vi "TEST - Sort Array.vi"(8 "error in (no error)":errorcluster) -> (0 "error out":errorcluster, 2 "Pass?":bool=TRUE)   [LabVIEW 2020]
doc: "This VI template can be used for the functional testing of VIs; this implementation includes handling for the testing of polymorphic VIs, and the polymorphic elements should be removed if not needed.\n\nCoded by Douglas A. Femec, January 24, 2006.\n\nCopyright (c) 2005-2006 MKS Instruments, Inc.\nAll rights reserved."
uses:
  TEST - Sort Array - Inputs.ctl
  Polymorphizer+ Data Type.ctl
  TEST - Sort Array - Outputs.ctl
  source/library/Sort Array/Sort 2D Array (EXT).vi
  source/library/Sort Array/Sort 1D Array (EXT).vi
  source/library/Sort Array/Sort 2D Array (DBL).vi
  source/library/Sort Array/Sort 1D Array (DBL).vi
  source/library/Sort Array/Sort 2D Array (SGL).vi
  source/library/Sort Array/Sort 1D Array (SGL).vi
  source/library/Sort Array/Sort 2D Array (I32).vi
  source/library/Sort Array/Sort 1D Array (I32).vi
  source/library/Sort Array/Sort 2D Array (I16).vi
  source/library/Sort Array/Sort 1D Array (I16).vi
  source/library/Sort Array/Sort 2D Array (I8).vi
  source/library/Sort Array/Sort 1D Array (I8).vi
  source/library/Sort Array/Sort 2D Array (I64).vi
  source/library/Sort Array/Sort 1D Array (I64).vi
  source/library/Sort Array/Sort 2D Array (U64).vi
  source/library/Sort Array/Sort 1D Array (U64).vi
  source/library/Sort Array/Sort 2D Array (U32).vi
  source/library/Sort Array/Sort 1D Array (U32).vi
  source/library/Sort Array/Sort 2D Array (U16).vi
  source/library/Sort Array/Sort 1D Array (U16).vi
  source/library/Sort Array/Sort 2D Array (U8).vi
  source/library/Sort Array/Sort 1D Array (U8).vi
  source/library/Sort Array/Sort 2D Array (CXT).vi
  source/library/Sort Array/Sort 1D Array (CXT).vi
  source/library/Sort Array/Sort 2D Array (CDB).vi
  source/library/Sort Array/Sort 1D Array (CDB).vi
  source/library/Sort Array/Sort 2D Array (CSG).vi
  source/library/Sort Array/Sort 1D Array (CSG).vi
  source/library/Sort Array/Sort 2D Array (String).vi
  source/library/Sort Array/Sort 1D Array (String).vi
  source/library/Sort Array/Sort 2D Array (Path).vi
  source/library/Sort Array/Sort 1D Array (Path).vi
  source/library/openg_array.lvlib
panel:
  out "Generated Outputs":T1[][](array[typedef]) {"1D Array" format="%.2f"; "2D Array" format="%.2f"}
  in  "Expected Outputs":T1[](array[typedef])=[{"Description"="Expect empty arrays", "1D Array"=[], "2D Array"=[], "1D Sorted Pointers"=[], "2D Sorted Pointers"=[], "Index Out of Range?"=FALSE, "Sort By in"=enum."row"}, {"Description"="Expect empty arrays", "1D Array"=[], "2D Array"=[], "1D Sorted Pointers"=[], "2D Sorted Pointers"=[], "Index Out of Range?"=FALSE, "Sort By in"=enum."row"}, {"Description"="Expect empty arrays", "1D Array"=[], "2D Array"=[], "1D Sorted Pointers"=[], "2D Sorted Pointers"=[], "Index Out of Range?"=FALSE, "Sort By in"=enum."row"}, {"Description"="Expect empty arrays", "1D Array"=[], "2D Array"=[], "1D Sorted Pointers"=[], "2D Sorted Pointers"=[], "Index Out of Range?"=FALSE, "Sort By in"=enum."column"}, {"Description"="Expect empty arrays", "1D Array"=[], "2D Array"=[], "1D Sorted Pointers"=[], "2D Sorted Pointers"=[], "Index Out of Range?"=FALSE, "Sort By in"=enum."column"}, {"Description"="Expect empty arrays", "1D Array"=[], "2D Array"=[], "1D Sorted Pointers"=[], "2D Sorted Pointers"=[], "Index Out of Range?"=FALSE, "Sort By in"=enum."column"}, {"Description"="Expect empty arrays", "1D Array"=[], "2D Array"=[], "1D Sorted Pointers"=[], "2D Sorted Pointers"=[], "Index Out of Range?"=FALSE, "Sort By in"=enum."row"}, {"Description"="Expect empty arrays", "1D Array"=[], "2D Array"=[], "1D Sorted Pointers"=[], "2D Sorted Pointers"=[], "Index Out of Range?"=FALSE, "Sort By in"=enum."row"}, {"Description"="Expect empty arrays", "1D Array"=[], "2D Array"=[], "1D Sorted Pointers"=[], "2D Sorted Pointers"=[], "Index Out of Range?"=FALSE, "Sort By in"=enum."row"}, {"Description"="Expect empty arrays", "1D Array"=[], "2D Array"=[], "1D Sorted Pointers"=[], "2D Sorted Pointers"=[], "Index Out of Range?"=FALSE, "Sort By in"=enum."column"}, {"Description"="Expect empty arrays", "1D Array"=[], "2D Array"=[], "1D Sorted Pointers"=[], "2D Sorted Pointers"=[], "Index Out of Range?"=FALSE, "Sort By in"=enum."column"}, {"Description"="Expect empty arrays", "1D Array"=[], "2D Array"=[], "1D Sorted Pointers"=[], "2D Sorted Pointers"=[], "Index Out of Range?"=FALSE, "Sort By in"=enum."column"}, {"Description"="Expect sorted in ascending order, 2D by row 0", "1D Array"=[0.0, 1.0, 2.0, 3.0, 4.0], "2D Array"=[[0.0, 5.0], [1.0, 6.0], [2.0, 7.0], [3.0, 8.0], [4.0, 9.0]], "1D Sorted Pointers"=[0, 1, 2, 3, 4], "2D Sorted Pointers"=[0, 1], "Index Out of Range?"=FALSE, "Sort By in"=enum."row"}, {"Description"="Expect sorted in ascending order, 2D by row 1", "1D Array"=[0.0, 1.0, 2.0, 3.0, 4.0], "2D Array"=[[0.0, 5.0], [1.0, 6.0], [2.0, 7.0], [3.0, 8.0], [4.0, 9.0]], "1D Sorted Pointers"=[0, 1, 2, 3, 4], "2D Sorted Pointers"=[0, 1], "Index Out of Range?"=FALSE, "Sort By in"=enum."row"}, {"Description"="Expect sorted in ascending order, 2D no row 5, so expect index out of range", "1D Array"=[0.0, 1.0, 2.0, 3.0, 4.0], "2D Array"=[], "1D Sorted Pointers"=[0, 1, 2, 3, 4], "2D Sorted Pointers"=[], "Index Out of Range?"=TRUE, "Sort By in"=enum."row"}, {"Description"="Expect sorted in ascending order, 2D by column 0", "1D Array"=[0.0, 1.0, 2.0, 3.0, 4.0], "2D Array"=[[0.0, 5.0], [1.0, 6.0], [2.0, 7.0], [3.0, 8.0], [4.0, 9.0]], "1D Sorted Pointers"=[0, 1, 2, 3, 4], "2D Sorted Pointers"=[0, 1, 2, 3, 4], "Index Out of Range?"=FALSE, "Sort By in"=enum."column"}, {"Description"="Expect sorted in ascending order, 2D by column 1", "1D Array"=[0.0, 1.0, 2.0, 3.0, 4.0], "2D Array"=[[0.0, 5.0], [1.0, 6.0], [2.0, 7.0], [3.0, 8.0], [4.0, 9.0]], "1D Sorted Pointers"=[0, 1, 2, 3, 4], "2D Sorted Pointers"=[0, 1, 2, 3, 4], "Index Out of Range?"=FALSE, "Sort By in"=enum."column"}, {"Description"="Expect sorted in ascending order, 2D no column 5, so expect index out of range", "1D Array"=[0.0, 1.0, 2.0, 3.0, 4.0], "2D Array"=[], "1D Sorted Pointers"=[0, 1, 2, 3, 4], "2D Sorted Pointers"=[], "Index Out of Range?"=TRUE, "Sort By in"=enum."column"}, {"Description"="Expect sorted in descending order, 2D by row 0", "1D Array"=[4.0, 3.0, 2.0, 1.0, 0.0], "2D Array"=[[5.0, 0.0], [6.0, 1.0], [7.0, 2.0], [8.0, 3.0], [9.0, 4.0]], "1D Sorted Pointers"=[4, 3, 2, 1, 0], "2D Sorted Pointers"=[1, 0], "Index Out of Range?"=FALSE, "Sort By in"=enum."row"}, {"Description"="Expect sorted in descending order, 2D by row 1", "1D Array"=[4.0, 3.0, 2.0, 1.0, 0.0], "2D Array"=[[5.0, 0.0], [6.0, 1.0], [7.0, 2.0], [8.0, 3.0], [9.0, 4.0]], "1D Sorted Pointers"=[4, 3, 2, 1, 0], "2D Sorted Pointers"=[1, 0], "Index Out of Range?"=FALSE, "Sort By in"=enum."row"}, {"Description"="Expect sorted in descending order, 2D no row 5, so expect index out of range", "1D Array"=[4.0, 3.0, 2.0, 1.0, 0.0], "2D Array"=[], "1D Sorted Pointers"=[4, 3, 2, 1, 0], "2D Sorted Pointers"=[], "Index Out of Range?"=TRUE, "Sort By in"=enum."row"}, {"Description"="Expect sorted in descending order, 2D by column 0", "1D Array"=[4.0, 3.0, 2.0, 1.0, 0.0], "2D Array"=[[4.0, 9.0], [3.0, 8.0], [2.0, 7.0], [1.0, 6.0], [0.0, 5.0]], "1D Sorted Pointers"=[4, 3, 2, 1, 0], "2D Sorted Pointers"=[4, 3, 2, 1, 0], "Index Out of Range?"=FALSE, "Sort By in"=enum."column"}, {"Description"="Expect sorted in descending order, 2D by column 1", "1D Array"=[4.0, 3.0, 2.0, 1.0, 0.0], "2D Array"=[[4.0, 9.0], [3.0, 8.0], [2.0, 7.0], [1.0, 6.0], [0.0, 5.0]], "1D Sorted Pointers"=[4, 3, 2, 1, 0], "2D Sorted Pointers"=[4, 3, 2, 1, 0], "Index Out of Range?"=FALSE, "Sort By in"=enum."column"}, {"Description"="Expect sorted in descending order, 2D no column 5, so expect index out of range", "1D Array"=[4.0, 3.0, 2.0, 1.0, 0.0], "2D Array"=[], "1D Sorted Pointers"=[4, 3, 2, 1, 0], "2D Sorted Pointers"=[], "Index Out of Range?"=TRUE, "Sort By in"=enum."column"}, {"Description"="Expect sorted in ascending order, 2D by row 0", "1D Array"=[0.0, 1.0, 2.0, 3.0, 4.0], "2D Array"=[[4.0, 9.0], [3.0, 8.0], [2.0, 7.0], [1.0, 6.0], [0.0, 5.0]], "1D Sorted Pointers"=[4, 3, 2, 1, 0], "2D Sorted Pointers"=[1, 0], "Index Out of Range?"=FALSE, "Sort By in"=enum."row"}, {"Description"="Expect sorted in ascending order, 2D by row 1", "1D Array"=[0.0, 1.0, 2.0, 3.0, 4.0], "2D Array"=[[4.0, 9.0], [3.0, 8.0], [2.0, 7.0], [1.0, 6.0], [0.0, 5.0]], "1D Sorted Pointers"=[4, 3, 2, 1, 0], "2D Sorted Pointers"=[1, 0], "Index Out of Range?"=FALSE, "Sort By in"=enum."row"}, {"Description"="Expect sorted in ascending order, 2D no row 5, so expect index out of range", "1D Array"=[0.0, 1.0, 2.0, 3.0, 4.0], "2D Array"=[], "1D Sorted Pointers"=[4, 3, 2, 1, 0], "2D Sorted Pointers"=[], "Index Out of Range?"=TRUE, "Sort By in"=enum."row"}, {"Description"="Expect sorted in descending order, 2D by column 0", "1D Array"=[0.0, 1.0, 2.0, 3.0, 4.0], "2D Array"=[[5.0, 0.0], [6.0, 1.0], [7.0, 2.0], [8.0, 3.0], [9.0, 4.0]], "1D Sorted Pointers"=[4, 3, 2, 1, 0], "2D Sorted Pointers"=[4, 3, 2, 1, 0], "Index Out of Range?"=FALSE, "Sort By in"=enum."column"}, {"Description"="Expect sorted in descending order, 2D by column 1", "1D Array"=[0.0, 1.0, 2.0, 3.0, 4.0], "2D Array"=[[5.0, 0.0], [6.0, 1.0], [7.0, 2.0], [8.0, 3.0], [9.0, 4.0]], "1D Sorted Pointers"=[4, 3, 2, 1, 0], "2D Sorted Pointers"=[4, 3, 2, 1, 0], "Index Out of Range?"=FALSE, "Sort By in"=enum."column"}, {"Description"="Expect sorted in descending order, 2D no column 5, so expect index out of range", "1D Array"=[0.0, 1.0, 2.0, 3.0, 4.0], "2D Array"=[], "1D Sorted Pointers"=[4, 3, 2, 1, 0], "2D Sorted Pointers"=[], "Index Out of Range?"=TRUE, "Sort By in"=enum."column"}, {"Description"="Expect sorted in descending order, 2D by row 0", "1D Array"=[4.0, 3.0, 2.0, 1.0, 0.0], "2D Array"=[[9.0, 4.0], [8.0, 3.0], [7.0, 2.0], [6.0, 1.0], [5.0, 0.0]], "1D Sorted Pointers"=[0, 1, 2, 3, 4], "2D Sorted Pointers"=[0, 1], "Index Out of Range?"=FALSE, "Sort By in"=enum."row"}, {"Description"="Expect sorted in descending order, 2D by row 1", "1D Array"=[4.0, 3.0, 2.0, 1.0, 0.0], "2D Array"=[[9.0, 4.0], [8.0, 3.0], [7.0, 2.0], [6.0, 1.0], [5.0, 0.0]], "1D Sorted Pointers"=[0, 1, 2, 3, 4], "2D Sorted Pointers"=[0, 1], "Index Out of Range?"=FALSE, "Sort By in"=enum."row"}, {"Description"="Expect sorted in descending order, 2D no row 5, so expect index out of range", "1D Array"=[4.0, 3.0, 2.0, 1.0, 0.0], "2D Array"=[], "1D Sorted Pointers"=[0, 1, 2, 3, 4], "2D Sorted Pointers"=[], "Index Out of Range?"=TRUE, "Sort By in"=enum."row"}, {"Description"="Expect sorted in descending order, 2D by column 0", "1D Array"=[4.0, 3.0, 2.0, 1.0, 0.0], "2D Array"=[[9.0, 4.0], [8.0, 3.0], [7.0, 2.0], [6.0, 1.0], [5.0, 0.0]], "1D Sorted Pointers"=[0, 1, 2, 3, 4], "2D Sorted Pointers"=[0, 1, 2, 3, 4], "Index Out of Range?"=FALSE, "Sort By in"=enum."column"}, {"Description"="Expect sorted in descending order, 2D by column 1", "1D Array"=[4.0, 3.0, 2.0, 1.0, 0.0], "2D Array"=[[9.0, 4.0], [8.0, 3.0], [7.0, 2.0], [6.0, 1.0], [5.0, 0.0]], "1D Sorted Pointers"=[0, 1, 2, 3, 4], "2D Sorted Pointers"=[0, 1, 2, 3, 4], "Index Out of Range?"=FALSE, "Sort By in"=enum."column"}, {"Description"="Expect sorted in descending order, 2D no column 5, so expect index out of range", "1D Array"=[4.0, 3.0, 2.0, 1.0, 0.0], "2D Array"=[], "1D Sorted Pointers"=[0, 1, 2, 3, 4], "2D Sorted Pointers"=[], "Index Out of Range?"=TRUE, "Sort By in"=enum."column"}, {"Description"="Expect sorted in ascending order, 2D by row 0", "1D Array"=[0.0, 1.0, 2.0, 3.0, 4.0], "2D Array"=[[3.0, 6.0], [2.0, 9.0], [0.0, 5.0], [4.0, 7.0], [1.0, 8.0]], "1D Sorted Pointers"=[2, 4, 1, 0, 3], "2D Sorted Pointers"=[0, 1], "Index Out of Range?"=FALSE, "Sort By in"=enum."row"}, {"Description"="Expect sorted in ascending order, 2D by row 1", "1D Array"=[0.0, 1.0, 2.0, 3.0, 4.0], "2D Array"=[[3.0, 6.0], [2.0, 9.0], [0.0, 5.0], [4.0, 7.0], [1.0, 8.0]], "1D Sorted Pointers"=[2, 4, 1, 0, 3], "2D Sorted Pointers"=[0, 1], "Index Out of Range?"=FALSE, "Sort By in"=enum."row"}, {"Description"="Expect sorted in ascending order, 2D no row 5, so expect index out of range", "1D Array"=[0.0, 1.0, 2.0, 3.0, 4.0], "2D Array"=[], "1D Sorted Pointers"=[2, 4, 1, 0, 3], "2D Sorted Pointers"=[], "Index Out of Range?"=TRUE, "Sort By in"=enum."row"}, {"Description"="Expect sorted in ascending order, 2D by column 0", "1D Array"=[0.0, 1.0, 2.0, 3.0, 4.0], "2D Array"=[[0.0, 5.0], [1.0, 8.0], [2.0, 9.0], [3.0, 6.0], [4.0, 7.0]], "1D Sorted Pointers"=[2, 4, 1, 0, 3], "2D Sorted Pointers"=[2, 4, 1, 0, 3], "Index Out of Range?"=FALSE, "Sort By in"=enum."column"}, {"Description"="Expect sorted in ascending order, 2D by column 1", "1D Array"=[0.0, 1.0, 2.0, 3.0, 4.0], "2D Array"=[[0.0, 5.0], [3.0, 6.0], [4.0, 7.0], [1.0, 8.0], [2.0, 9.0]], "1D Sorted Pointers"=[2, 4, 1, 0, 3], "2D Sorted Pointers"=[2, 0, 3, 4, 1], "Index Out of Range?"=FALSE, "Sort By in"=enum."column"}, {"Description"="Expect sorted in ascending order, 2D no column 5, so expect index out of range", "1D Array"=[0.0, 1.0, 2.0, 3.0, 4.0], "2D Array"=[], "1D Sorted Pointers"=[2, 4, 1, 0, 3], "2D Sorted Pointers"=[], "Index Out of Range?"=TRUE, "Sort By in"=enum."column"}, {"Description"="Expect sorted in descending order, 2D by row 0", "1D Array"=[4.0, 3.0, 2.0, 1.0, 0.0], "2D Array"=[[6.0, 3.0], [9.0, 2.0], [5.0, 0.0], [7.0, 4.0], [8.0, 1.0]], "1D Sorted Pointers"=[3, 0, 1, 4, 2], "2D Sorted Pointers"=[1, 0], "Index Out of Range?"=FALSE, "Sort By in"=enum."row"}, {"Description"="Expect sorted in descending order, 2D by row 1", "1D Array"=[4.0, 3.0, 2.0, 1.0, 0.0], "2D Array"=[[6.0, 3.0], [9.0, 2.0], [5.0, 0.0], [7.0, 4.0], [8.0, 1.0]], "1D Sorted Pointers"=[3, 0, 1, 4, 2], "2D Sorted Pointers"=[1, 0], "Index Out of Range?"=FALSE, "Sort By in"=enum."row"}, {"Description"="Expect sorted in descending order, 2D no row 5, so expect index out of range", "1D Array"=[4.0, 3.0, 2.0, 1.0, 0.0], "2D Array"=[], "1D Sorted Pointers"=[3, 0, 1, 4, 2], "2D Sorted Pointers"=[], "Index Out of Range?"=TRUE, "Sort By in"=enum."row"}, {"Description"="Expect sorted in descending order, 2D by column 0", "1D Array"=[4.0, 3.0, 2.0, 1.0, 0.0], "2D Array"=[[4.0, 7.0], [3.0, 6.0], [2.0, 9.0], [1.0, 8.0], [0.0, 5.0]], "1D Sorted Pointers"=[3, 0, 1, 4, 2], "2D Sorted Pointers"=[3, 0, 1, 4, 2], "Index Out of Range?"=FALSE, "Sort By in"=enum."column"}, {"Description"="Expect sorted in descending order, 2D by column 1", "1D Array"=[4.0, 3.0, 2.0, 1.0, 0.0], "2D Array"=[[2.0, 9.0], [1.0, 8.0], [4.0, 7.0], [3.0, 6.0], [0.0, 5.0]], "1D Sorted Pointers"=[3, 0, 1, 4, 2], "2D Sorted Pointers"=[1, 4, 3, 0, 2], "Index Out of Range?"=FALSE, "Sort By in"=enum."column"}, {"Description"="Expect sorted in ascending order, 2D no column 5, so expect index out of range", "1D Array"=[4.0, 3.0, 2.0, 1.0, 0.0], "2D Array"=[], "1D Sorted Pointers"=[3, 0, 1, 4, 2], "2D Sorted Pointers"=[], "Index Out of Range?"=TRUE, "Sort By in"=enum."column"}] {"1D Array" format="%.2f"; "2D Array" format="%.2f"}
  in  "Inputs":T2[](array[typedef])=[{"Description"="Empty arrays, ascending, 2D by row 0", "Data Types to Test"=[enum."EXT", enum."DBL", enum."SGL", enum."I32", enum."I16", enum."I8", enum."U32", enum."U16", enum."U8", enum."CXT", enum."CDB", enum."CSG", enum."String", enum."Path", enum."I64", enum."U64"], "1D Array"=[], "2D Array"=[], "Order"=enum."ascending", "Sort By in"=enum."row", "Column/Row to Sort By"=0}, {"Description"="Empty arrays, ascending, 2D by row 1", "Data Types to Test"=[enum."EXT", enum."DBL", enum."SGL", enum."I32", enum."I16", enum."I8", enum."U32", enum."U16", enum."U8", enum."CXT", enum."CDB", enum."CSG", enum."String", enum."Path", enum."I64", enum."U64"], "1D Array"=[], "2D Array"=[], "Order"=enum."ascending", "Sort By in"=enum."row", "Column/Row to Sort By"=1}, {"Description"="Empty arrays, ascending, 2D by row 5", "Data Types to Test"=[enum."EXT", enum."DBL", enum."SGL", enum."I32", enum."I16", enum."I8", enum."U32", enum."U16", enum."U8", enum."CXT", enum."CDB", enum."CSG", enum."String", enum."Path", enum."I64", enum."U64"], "1D Array"=[], "2D Array"=[], "Order"=enum."ascending", "Sort By in"=enum."row", "Column/Row to Sort By"=5}, {"Description"="Empty arrays, ascending, 2D by column 0", "Data Types to Test"=[enum."EXT", enum."DBL", enum."SGL", enum."I32", enum."I16", enum."I8", enum."U32", enum."U16", enum."U8", enum."CXT", enum."CDB", enum."CSG", enum."String", enum."Path", enum."I64", enum."U64"], "1D Array"=[], "2D Array"=[], "Order"=enum."ascending", "Sort By in"=enum."column", "Column/Row to Sort By"=0}, {"Description"="Empty arrays, ascending, 2D by column 1", "Data Types to Test"=[enum."EXT", enum."DBL", enum."SGL", enum."I32", enum."I16", enum."I8", enum."U32", enum."U16", enum."U8", enum."CXT", enum."CDB", enum."CSG", enum."String", enum."Path", enum."I64", enum."U64"], "1D Array"=[], "2D Array"=[], "Order"=enum."ascending", "Sort By in"=enum."column", "Column/Row to Sort By"=1}, {"Description"="Empty arrays, ascending, 2D by column 5", "Data Types to Test"=[enum."EXT", enum."DBL", enum."SGL", enum."I32", enum."I16", enum."I8", enum."U32", enum."U16", enum."U8", enum."CXT", enum."CDB", enum."CSG", enum."String", enum."Path", enum."I64", enum."U64"], "1D Array"=[], "2D Array"=[], "Order"=enum."ascending", "Sort By in"=enum."column", "Column/Row to Sort By"=5}, {"Description"="Empty arrays, descending, 2D by row 0", "Data Types to Test"=[enum."EXT", enum."DBL", enum."SGL", enum."I32", enum."I16", enum."I8", enum."U32", enum."U16", enum."U8", enum."CXT", enum."CDB", enum."CSG", enum."String", enum."Path", enum."I64", enum."U64"], "1D Array"=[], "2D Array"=[], "Order"=enum."descending", "Sort By in"=enum."row", "Column/Row to Sort By"=0}, {"Description"="Empty arrays, descending, 2D by row 1", "Data Types to Test"=[enum."EXT", enum."DBL", enum."SGL", enum."I32", enum."I16", enum."I8", enum."U32", enum."U16", enum."U8", enum."CXT", enum."CDB", enum."CSG", enum."String", enum."Path", enum."I64", enum."U64"], "1D Array"=[], "2D Array"=[], "Order"=enum."descending", "Sort By in"=enum."row", "Column/Row to Sort By"=1}, {"Description"="Empty arrays, descending, 2D by row 5", "Data Types to Test"=[enum."EXT", enum."DBL", enum."SGL", enum."I32", enum."I16", enum."I8", enum."U32", enum."U16", enum."U8", enum."CXT", enum."CDB", enum."CSG", enum."String", enum."Path", enum."I64", enum."U64"], "1D Array"=[], "2D Array"=[], "Order"=enum."descending", "Sort By in"=enum."row", "Column/Row to Sort By"=5}, {"Description"="Empty arrays, descending, 2D by column 0", "Data Types to Test"=[enum."EXT", enum."DBL", enum."SGL", enum."I32", enum."I16", enum."I8", enum."U32", enum."U16", enum."U8", enum."CXT", enum."CDB", enum."CSG", enum."String", enum."Path", enum."I64", enum."U64"], "1D Array"=[], "2D Array"=[], "Order"=enum."descending", "Sort By in"=enum."column", "Column/Row to Sort By"=0}, {"Description"="Empty arrays, descending, 2D by column 1", "Data Types to Test"=[enum."EXT", enum."DBL", enum."SGL", enum."I32", enum."I16", enum."I8", enum."U32", enum."U16", enum."U8", enum."CXT", enum."CDB", enum."CSG", enum."String", enum."Path", enum."I64", enum."U64"], "1D Array"=[], "2D Array"=[], "Order"=enum."descending", "Sort By in"=enum."column", "Column/Row to Sort By"=1}, {"Description"="Empty arrays, descending, 2D by column 5", "Data Types to Test"=[enum."EXT", enum."DBL", enum."SGL", enum."I32", enum."I16", enum."I8", enum."U32", enum."U16", enum."U8", enum."CXT", enum."CDB", enum."CSG", enum."String", enum."Path", enum."I64", enum."U64"], "1D Array"=[], "2D Array"=[], "Order"=enum."descending", "Sort By in"=enum."column", "Column/Row to Sort By"=5}, {"Description"="Already sorted in ascending order, ascending, 2D by row 0", "Data Types to Test"=[enum."EXT", enum."DBL", enum."SGL", enum."I32", enum."I16", enum."I8", enum."U32", enum."U16", enum."U8", enum."CXT", enum."CDB", enum."CSG", enum."String", enum."Path", enum."I64", enum."U64"], "1D Array"=[0.0, 1.0, 2.0, 3.0, 4.0], "2D Array"=[[0.0, 5.0], [1.0, 6.0], [2.0, 7.0], [3.0, 8.0], [4.0, 9.0]], "Order"=enum."ascending", "Sort By in"=enum."row", "Column/Row to Sort By"=0}, {"Description"="Already sorted in ascending order, ascending, 2D by row 1", "Data Types to Test"=[enum."EXT", enum."DBL", enum."SGL", enum."I32", enum."I16", enum."I8", enum."U32", enum."U16", enum."U8", enum."CXT", enum."CDB", enum."CSG", enum."String", enum."Path", enum."I64", enum."U64"], "1D Array"=[0.0, 1.0, 2.0, 3.0, 4.0], "2D Array"=[[0.0, 5.0], [1.0, 6.0], [2.0, 7.0], [3.0, 8.0], [4.0, 9.0]], "Order"=enum."ascending", "Sort By in"=enum."row", "Column/Row to Sort By"=1}, {"Description"="Already sorted in ascending order, ascending, 2D by row 5", "Data Types to Test"=[enum."EXT", enum."DBL", enum."SGL", enum."I32", enum."I16", enum."I8", enum."U32", enum."U16", enum."U8", enum."CXT", enum."CDB", enum."CSG", enum."String", enum."Path", enum."I64", enum."U64"], "1D Array"=[0.0, 1.0, 2.0, 3.0, 4.0], "2D Array"=[[0.0, 5.0], [1.0, 6.0], [2.0, 7.0], [3.0, 8.0], [4.0, 9.0]], "Order"=enum."ascending", "Sort By in"=enum."row", "Column/Row to Sort By"=5}, {"Description"="Already sorted in ascending order, ascending, 2D by column 0", "Data Types to Test"=[enum."EXT", enum."DBL", enum."SGL", enum."I32", enum."I16", enum."I8", enum."U32", enum."U16", enum."U8", enum."CXT", enum."CDB", enum."CSG", enum."String", enum."Path", enum."I64", enum."U64"], "1D Array"=[0.0, 1.0, 2.0, 3.0, 4.0], "2D Array"=[[0.0, 5.0], [1.0, 6.0], [2.0, 7.0], [3.0, 8.0], [4.0, 9.0]], "Order"=enum."ascending", "Sort By in"=enum."column", "Column/Row to Sort By"=0}, {"Description"="Already sorted in ascending order, ascending, 2D by column 1", "Data Types to Test"=[enum."EXT", enum."DBL", enum."SGL", enum."I32", enum."I16", enum."I8", enum."U32", enum."U16", enum."U8", enum."CXT", enum."CDB", enum."CSG", enum."String", enum."Path", enum."I64", enum."U64"], "1D Array"=[0.0, 1.0, 2.0, 3.0, 4.0], "2D Array"=[[0.0, 5.0], [1.0, 6.0], [2.0, 7.0], [3.0, 8.0], [4.0, 9.0]], "Order"=enum."ascending", "Sort By in"=enum."column", "Column/Row to Sort By"=1}, {"Description"="Already sorted in ascending order, ascending, 2D by column 5", "Data Types to Test"=[enum."EXT", enum."DBL", enum."SGL", enum."I32", enum."I16", enum."I8", enum."U32", enum."U16", enum."U8", enum."CXT", enum."CDB", enum."CSG", enum."String", enum."Path", enum."I64", enum."U64"], "1D Array"=[0.0, 1.0, 2.0, 3.0, 4.0], "2D Array"=[[0.0, 5.0], [1.0, 6.0], [2.0, 7.0], [3.0, 8.0], [4.0, 9.0]], "Order"=enum."ascending", "Sort By in"=enum."column", "Column/Row to Sort By"=5}, {"Description"="Already sorted in ascending order, descending, 2D by row 0", "Data Types to Test"=[enum."EXT", enum."DBL", enum."SGL", enum."I32", enum."I16", enum."I8", enum."U32", enum."U16", enum."U8", enum."CXT", enum."CDB", enum."CSG", enum."String", enum."Path", enum."I64", enum."U64"], "1D Array"=[0.0, 1.0, 2.0, 3.0, 4.0], "2D Array"=[[0.0, 5.0], [1.0, 6.0], [2.0, 7.0], [3.0, 8.0], [4.0, 9.0]], "Order"=enum."descending", "Sort By in"=enum."row", "Column/Row to Sort By"=0}, {"Description"="Already sorted in ascending order, descending, 2D by row 1", "Data Types to Test"=[enum."EXT", enum."DBL", enum."SGL", enum."I32", enum."I16", enum."I8", enum."U32", enum."U16", enum."U8", enum."CXT", enum."CDB", enum."CSG", enum."String", enum."Path", enum."I64", enum."U64"], "1D Array"=[0.0, 1.0, 2.0, 3.0, 4.0], "2D Array"=[[0.0, 5.0], [1.0, 6.0], [2.0, 7.0], [3.0, 8.0], [4.0, 9.0]], "Order"=enum."descending", "Sort By in"=enum."row", "Column/Row to Sort By"=1}, {"Description"="Already sorted in ascending order, descending, 2D by row 5", "Data Types to Test"=[enum."EXT", enum."DBL", enum."SGL", enum."I32", enum."I16", enum."I8", enum."U32", enum."U16", enum."U8", enum."CXT", enum."CDB", enum."CSG", enum."String", enum."Path", enum."I64", enum."U64"], "1D Array"=[0.0, 1.0, 2.0, 3.0, 4.0], "2D Array"=[[0.0, 5.0], [1.0, 6.0], [2.0, 7.0], [3.0, 8.0], [4.0, 9.0]], "Order"=enum."descending", "Sort By in"=enum."row", "Column/Row to Sort By"=5}, {"Description"="Already sorted in ascending order, descending, 2D by column 0", "Data Types to Test"=[enum."EXT", enum."DBL", enum."SGL", enum."I32", enum."I16", enum."I8", enum."U32", enum."U16", enum."U8", enum."CXT", enum."CDB", enum."CSG", enum."String", enum."Path", enum."I64", enum."U64"], "1D Array"=[0.0, 1.0, 2.0, 3.0, 4.0], "2D Array"=[[0.0, 5.0], [1.0, 6.0], [2.0, 7.0], [3.0, 8.0], [4.0, 9.0]], "Order"=enum."descending", "Sort By in"=enum."column", "Column/Row to Sort By"=0}, {"Description"="Already sorted in ascending order, descending, 2D by column 1", "Data Types to Test"=[enum."EXT", enum."DBL", enum."SGL", enum."I32", enum."I16", enum."I8", enum."U32", enum."U16", enum."U8", enum."CXT", enum."CDB", enum."CSG", enum."String", enum."Path", enum."I64", enum."U64"], "1D Array"=[0.0, 1.0, 2.0, 3.0, 4.0], "2D Array"=[[0.0, 5.0], [1.0, 6.0], [2.0, 7.0], [3.0, 8.0], [4.0, 9.0]], "Order"=enum."descending", "Sort By in"=enum."column", "Column/Row to Sort By"=1}, {"Description"="Already sorted in ascending order, descending, 2D by column 5", "Data Types to Test"=[enum."EXT", enum."DBL", enum."SGL", enum."I32", enum."I16", enum."I8", enum."U32", enum."U16", enum."U8", enum."CXT", enum."CDB", enum."CSG", enum."String", enum."Path", enum."I64", enum."U64"], "1D Array"=[0.0, 1.0, 2.0, 3.0, 4.0], "2D Array"=[[0.0, 5.0], [1.0, 6.0], [2.0, 7.0], [3.0, 8.0], [4.0, 9.0]], "Order"=enum."descending", "Sort By in"=enum."column", "Column/Row to Sort By"=5}, {"Description"="Already sorted in descending order, ascending, 2D by row 0", "Data Types to Test"=[enum."EXT", enum."DBL", enum."SGL", enum."I32", enum."I16", enum."I8", enum."U32", enum."U16", enum."U8", enum."CXT", enum."CDB", enum."CSG", enum."String", enum."Path", enum."I64", enum."U64"], "1D Array"=[4.0, 3.0, 2.0, 1.0, 0.0], "2D Array"=[[9.0, 4.0], [8.0, 3.0], [7.0, 2.0], [6.0, 1.0], [5.0, 0.0]], "Order"=enum."ascending", "Sort By in"=enum."row", "Column/Row to Sort By"=0}, {"Description"="Already sorted in descending order, ascending, 2D by row 1", "Data Types to Test"=[enum."EXT", enum."DBL", enum."SGL", enum."I32", enum."I16", enum."I8", enum."U32", enum."U16", enum."U8", enum."CXT", enum."CDB", enum."CSG", enum."String", enum."Path", enum."I64", enum."U64"], "1D Array"=[4.0, 3.0, 2.0, 1.0, 0.0], "2D Array"=[[9.0, 4.0], [8.0, 3.0], [7.0, 2.0], [6.0, 1.0], [5.0, 0.0]], "Order"=enum."ascending", "Sort By in"=enum."row", "Column/Row to Sort By"=1}, {"Description"="Already sorted in descending order, ascending, 2D by row 5", "Data Types to Test"=[enum."EXT", enum."DBL", enum."SGL", enum."I32", enum."I16", enum."I8", enum."U32", enum."U16", enum."U8", enum."CXT", enum."CDB", enum."CSG", enum."String", enum."Path", enum."I64", enum."U64"], "1D Array"=[4.0, 3.0, 2.0, 1.0, 0.0], "2D Array"=[[9.0, 4.0], [8.0, 3.0], [7.0, 2.0], [6.0, 2.0], [5.0, 1.0]], "Order"=enum."ascending", "Sort By in"=enum."row", "Column/Row to Sort By"=5}, {"Description"="Already sorted in descending order, ascending, 2D by column 0", "Data Types to Test"=[enum."EXT", enum."DBL", enum."SGL", enum."I32", enum."I16", enum."I8", enum."U32", enum."U16", enum."U8", enum."CXT", enum."CDB", enum."CSG", enum."String", enum."Path", enum."I64", enum."U64"], "1D Array"=[4.0, 3.0, 2.0, 1.0, 0.0], "2D Array"=[[9.0, 4.0], [8.0, 3.0], [7.0, 2.0], [6.0, 1.0], [5.0, 0.0]], "Order"=enum."ascending", "Sort By in"=enum."column", "Column/Row to Sort By"=0}, {"Description"="Already sorted in descending order, ascending, 2D by column 1", "Data Types to Test"=[enum."EXT", enum."DBL", enum."SGL", enum."I32", enum."I16", enum."I8", enum."U32", enum."U16", enum."U8", enum."CXT", enum."CDB", enum."CSG", enum."String", enum."Path", enum."I64", enum."U64"], "1D Array"=[4.0, 3.0, 2.0, 1.0, 0.0], "2D Array"=[[9.0, 4.0], [8.0, 3.0], [7.0, 2.0], [6.0, 1.0], [5.0, 0.0]], "Order"=enum."ascending", "Sort By in"=enum."column", "Column/Row to Sort By"=1}, {"Description"="Already sorted in descending order, ascending, 2D by column 5", "Data Types to Test"=[enum."EXT", enum."DBL", enum."SGL", enum."I32", enum."I16", enum."I8", enum."U32", enum."U16", enum."U8", enum."CXT", enum."CDB", enum."CSG", enum."String", enum."Path", enum."I64", enum."U64"], "1D Array"=[4.0, 3.0, 2.0, 1.0, 0.0], "2D Array"=[[9.0, 4.0], [8.0, 3.0], [7.0, 2.0], [6.0, 2.0], [5.0, 1.0]], "Order"=enum."ascending", "Sort By in"=enum."column", "Column/Row to Sort By"=5}, {"Description"="Already sorted in descending order, descending, 2D by row 0", "Data Types to Test"=[enum."EXT", enum."DBL", enum."SGL", enum."I32", enum."I16", enum."I8", enum."U32", enum."U16", enum."U8", enum."CXT", enum."CDB", enum."CSG", enum."String", enum."Path", enum."I64", enum."U64"], "1D Array"=[4.0, 3.0, 2.0, 1.0, 0.0], "2D Array"=[[9.0, 4.0], [8.0, 3.0], [7.0, 2.0], [6.0, 1.0], [5.0, 0.0]], "Order"=enum."descending", "Sort By in"=enum."row", "Column/Row to Sort By"=0}, {"Description"="Already sorted in descending order, descending, 2D by row 1", "Data Types to Test"=[enum."EXT", enum."DBL", enum."SGL", enum."I32", enum."I16", enum."I8", enum."U32", enum."U16", enum."U8", enum."CXT", enum."CDB", enum."CSG", enum."String", enum."Path", enum."I64", enum."U64"], "1D Array"=[4.0, 3.0, 2.0, 1.0, 0.0], "2D Array"=[[9.0, 4.0], [8.0, 3.0], [7.0, 2.0], [6.0, 1.0], [5.0, 0.0]], "Order"=enum."descending", "Sort By in"=enum."row", "Column/Row to Sort By"=1}, {"Description"="Already sorted in descending order, descending, 2D by row 5", "Data Types to Test"=[enum."EXT", enum."DBL", enum."SGL", enum."I32", enum."I16", enum."I8", enum."U32", enum."U16", enum."U8", enum."CXT", enum."CDB", enum."CSG", enum."String", enum."Path", enum."I64", enum."U64"], "1D Array"=[4.0, 3.0, 2.0, 1.0, 0.0], "2D Array"=[[9.0, 4.0], [8.0, 3.0], [7.0, 2.0], [6.0, 2.0], [5.0, 1.0]], "Order"=enum."descending", "Sort By in"=enum."row", "Column/Row to Sort By"=5}, {"Description"="Already sorted in descending order, descending, 2D by column 0", "Data Types to Test"=[enum."EXT", enum."DBL", enum."SGL", enum."I32", enum."I16", enum."I8", enum."U32", enum."U16", enum."U8", enum."CXT", enum."CDB", enum."CSG", enum."String", enum."Path", enum."I64", enum."U64"], "1D Array"=[4.0, 3.0, 2.0, 1.0, 0.0], "2D Array"=[[9.0, 4.0], [8.0, 3.0], [7.0, 2.0], [6.0, 1.0], [5.0, 0.0]], "Order"=enum."descending", "Sort By in"=enum."column", "Column/Row to Sort By"=0}, {"Description"="Already sorted in descending order, descending, 2D by column 1", "Data Types to Test"=[enum."EXT", enum."DBL", enum."SGL", enum."I32", enum."I16", enum."I8", enum."U32", enum."U16", enum."U8", enum."CXT", enum."CDB", enum."CSG", enum."String", enum."Path", enum."I64", enum."U64"], "1D Array"=[4.0, 3.0, 2.0, 1.0, 0.0], "2D Array"=[[9.0, 4.0], [8.0, 3.0], [7.0, 2.0], [6.0, 1.0], [5.0, 0.0]], "Order"=enum."descending", "Sort By in"=enum."column", "Column/Row to Sort By"=1}, {"Description"="Already sorted in descending order, descending, 2D by column 5", "Data Types to Test"=[enum."EXT", enum."DBL", enum."SGL", enum."I32", enum."I16", enum."I8", enum."U32", enum."U16", enum."U8", enum."CXT", enum."CDB", enum."CSG", enum."String", enum."Path", enum."I64", enum."U64"], "1D Array"=[4.0, 3.0, 2.0, 1.0, 0.0], "2D Array"=[[9.0, 4.0], [8.0, 3.0], [7.0, 2.0], [6.0, 1.0], [5.0, 0.0]], "Order"=enum."descending", "Sort By in"=enum."column", "Column/Row to Sort By"=5}, {"Description"="Not sorted, ascending, 2D by row 0", "Data Types to Test"=[enum."EXT", enum."DBL", enum."SGL", enum."I32", enum."I16", enum."I8", enum."U32", enum."U16", enum."U8", enum."CXT", enum."CDB", enum."CSG", enum."String", enum."Path", enum."I64", enum."U64"], "1D Array"=[3.0, 2.0, 0.0, 4.0, 1.0], "2D Array"=[[3.0, 6.0], [2.0, 9.0], [0.0, 5.0], [4.0, 7.0], [1.0, 8.0]], "Order"=enum."ascending", "Sort By in"=enum."row", "Column/Row to Sort By"=0}, {"Description"="Not sorted, ascending, 2D by row 1", "Data Types to Test"=[enum."EXT", enum."DBL", enum."SGL", enum."I32", enum."I16", enum."I8", enum."U32", enum."U16", enum."U8", enum."CXT", enum."CDB", enum."CSG", enum."String", enum."Path", enum."I64", enum."U64"], "1D Array"=[3.0, 2.0, 0.0, 4.0, 1.0], "2D Array"=[[3.0, 6.0], [2.0, 9.0], [0.0, 5.0], [4.0, 7.0], [1.0, 8.0]], "Order"=enum."ascending", "Sort By in"=enum."row", "Column/Row to Sort By"=1}, {"Description"="Not sorted, ascending, 2D by row 5", "Data Types to Test"=[enum."EXT", enum."DBL", enum."SGL", enum."I32", enum."I16", enum."I8", enum."U32", enum."U16", enum."U8", enum."CXT", enum."CDB", enum."CSG", enum."String", enum."Path", enum."I64", enum."U64"], "1D Array"=[3.0, 2.0, 0.0, 4.0, 1.0], "2D Array"=[[3.0, 6.0], [2.0, 9.0], [0.0, 5.0], [4.0, 7.0], [1.0, 8.0]], "Order"=enum."ascending", "Sort By in"=enum."row", "Column/Row to Sort By"=5}, {"Description"="Not sorted, ascending, 2D by column 0", "Data Types to Test"=[enum."EXT", enum."DBL", enum."SGL", enum."I32", enum."I16", enum."I8", enum."U32", enum."U16", enum."U8", enum."CXT", enum."CDB", enum."CSG", enum."String", enum."Path", enum."I64", enum."U64"], "1D Array"=[3.0, 2.0, 0.0, 4.0, 1.0], "2D Array"=[[3.0, 6.0], [2.0, 9.0], [0.0, 5.0], [4.0, 7.0], [1.0, 8.0]], "Order"=enum."ascending", "Sort By in"=enum."column", "Column/Row to Sort By"=0}, {"Description"="Not sorted, ascending, 2D by column 1", "Data Types to Test"=[enum."EXT", enum."DBL", enum."SGL", enum."I32", enum."I16", enum."I8", enum."U32", enum."U16", enum."U8", enum."CXT", enum."CDB", enum."CSG", enum."String", enum."Path", enum."I64", enum."U64"], "1D Array"=[3.0, 2.0, 0.0, 4.0, 1.0], "2D Array"=[[3.0, 6.0], [2.0, 9.0], [0.0, 5.0], [4.0, 7.0], [1.0, 8.0]], "Order"=enum."ascending", "Sort By in"=enum."column", "Column/Row to Sort By"=1}, {"Description"="Not sorted, ascending, 2D by column 5", "Data Types to Test"=[enum."EXT", enum."DBL", enum."SGL", enum."I32", enum."I16", enum."I8", enum."U32", enum."U16", enum."U8", enum."CXT", enum."CDB", enum."CSG", enum."String", enum."Path", enum."I64", enum."U64"], "1D Array"=[3.0, 2.0, 0.0, 4.0, 1.0], "2D Array"=[[3.0, 6.0], [2.0, 9.0], [0.0, 5.0], [4.0, 7.0], [1.0, 8.0]], "Order"=enum."ascending", "Sort By in"=enum."column", "Column/Row to Sort By"=5}, {"Description"="Not sorted, descending, 2D by row 0", "Data Types to Test"=[enum."EXT", enum."DBL", enum."SGL", enum."I32", enum."I16", enum."I8", enum."U32", enum."U16", enum."U8", enum."CXT", enum."CDB", enum."CSG", enum."String", enum."Path", enum."I64", enum."U64"], "1D Array"=[3.0, 2.0, 0.0, 4.0, 1.0], "2D Array"=[[3.0, 6.0], [2.0, 9.0], [0.0, 5.0], [4.0, 7.0], [1.0, 8.0]], "Order"=enum."descending", "Sort By in"=enum."row", "Column/Row to Sort By"=0}, {"Description"="Not sorted, descending, 2D by row 1", "Data Types to Test"=[enum."EXT", enum."DBL", enum."SGL", enum."I32", enum."I16", enum."I8", enum."U32", enum."U16", enum."U8", enum."CXT", enum."CDB", enum."CSG", enum."String", enum."Path", enum."I64", enum."U64"], "1D Array"=[3.0, 2.0, 0.0, 4.0, 1.0], "2D Array"=[[3.0, 6.0], [2.0, 9.0], [0.0, 5.0], [4.0, 7.0], [1.0, 8.0]], "Order"=enum."descending", "Sort By in"=enum."row", "Column/Row to Sort By"=1}, {"Description"="Not sorted, descending, 2D by row 5", "Data Types to Test"=[enum."EXT", enum."DBL", enum."SGL", enum."I32", enum."I16", enum."I8", enum."U32", enum."U16", enum."U8", enum."CXT", enum."CDB", enum."CSG", enum."String", enum."Path", enum."I64", enum."U64"], "1D Array"=[3.0, 2.0, 0.0, 4.0, 1.0], "2D Array"=[[3.0, 6.0], [2.0, 9.0], [0.0, 5.0], [4.0, 7.0], [1.0, 8.0]], "Order"=enum."descending", "Sort By in"=enum."row", "Column/Row to Sort By"=5}, {"Description"="Not sorted, descending, 2D by column 0", "Data Types to Test"=[enum."EXT", enum."DBL", enum."SGL", enum."I32", enum."I16", enum."I8", enum."U32", enum."U16", enum."U8", enum."CXT", enum."CDB", enum."CSG", enum."String", enum."Path", enum."I64", enum."U64"], "1D Array"=[3.0, 2.0, 0.0, 4.0, 1.0], "2D Array"=[[3.0, 6.0], [2.0, 9.0], [0.0, 5.0], [4.0, 7.0], [1.0, 8.0]], "Order"=enum."descending", "Sort By in"=enum."column", "Column/Row to Sort By"=0}, {"Description"="Not sorted, descending, 2D by column 1", "Data Types to Test"=[enum."EXT", enum."DBL", enum."SGL", enum."I32", enum."I16", enum."I8", enum."U32", enum."U16", enum."U8", enum."CXT", enum."CDB", enum."CSG", enum."String", enum."Path", enum."I64", enum."U64"], "1D Array"=[3.0, 2.0, 0.0, 4.0, 1.0], "2D Array"=[[3.0, 6.0], [2.0, 9.0], [0.0, 5.0], [4.0, 7.0], [1.0, 8.0]], "Order"=enum."descending", "Sort By in"=enum."column", "Column/Row to Sort By"=1}, {"Description"="Not sorted, descending, 2D by column 5", "Data Types to Test"=[enum."EXT", enum."DBL", enum."SGL", enum."I32", enum."I16", enum."I8", enum."U32", enum."U16", enum."U8", enum."CXT", enum."CDB", enum."CSG", enum."String", enum."Path", enum."I64", enum."U64"], "1D Array"=[3.0, 2.0, 0.0, 4.0, 1.0], "2D Array"=[[3.0, 6.0], [2.0, 9.0], [0.0, 5.0], [4.0, 7.0], [1.0, 8.0]], "Order"=enum."descending", "Sort By in"=enum."column", "Column/Row to Sort By"=5}] {"1D Array" format="%.2f"; "2D Array" format="%.2f"}
  # "Copyright (c) 2005-2006 MKS Instruments, Inc.\nAll rights reserved."
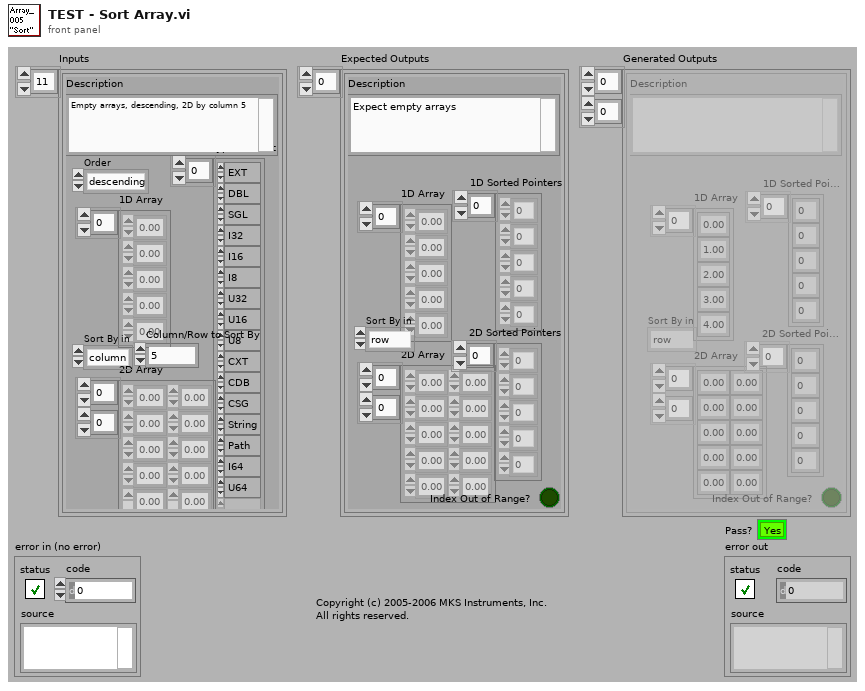
[diagram p1: front panel]
types:
  T1 = typedef "TEST - Sort Array - Outputs.ctl" = cluster{"Description":string, "1D Array":sgl[], "2D Array":sgl[][], "1D Sorted Pointers":i32[], "2D Sorted Pointers":i32[], "Index Out of Range?":bool, "Sort By in":enum16{"row", "column"}}
  T2 = typedef "TEST - Sort Array - Inputs.ctl" = cluster{"Description":string, "Data Types to Test":T3[], "1D Array":sgl[], "2D Array":sgl[][], "Order":enum16{"ascending", "descending"}, "Sort By in":enum16{"row", "column"}, "Column/Row to Sort By":u32}
  T3 = typedef "Polymorphizer+ Data Type.ctl" = enum16{"EXT", "DBL", "SGL", "I32", "I16", "I8", "U32", "U16", "U8", "CXT", "CDB", "CSG", "Boolean", "String", "Path", "Variant", "CTL-REF", "GEN-REF", "GObj-REF", "VI-REF", "ENUM", "ERR", "FILE-REF", "MENU-REF", "MENU-RING", "PICT-RING", "TXT&PICT-RING", "TXT-RING", "I64", "U64", "LabVIEW Object"}
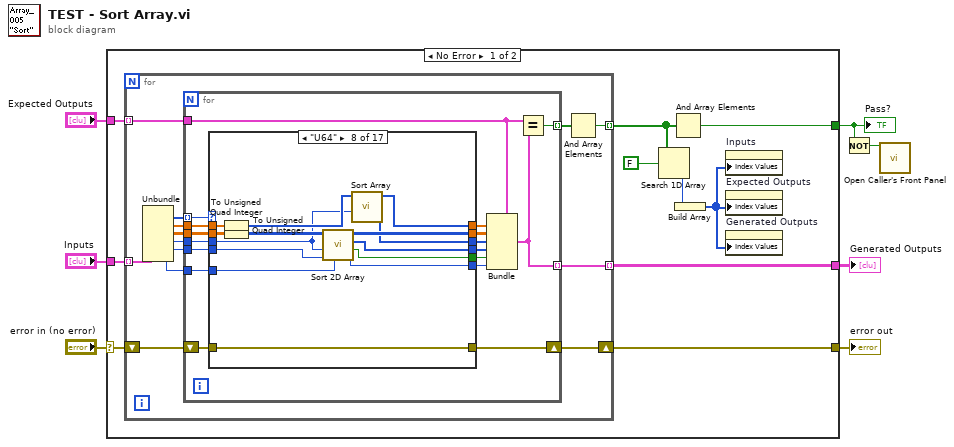
[diagram p0: block diagram]
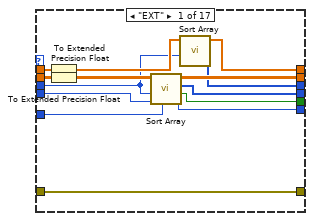
[diagram p2: hidden frame]
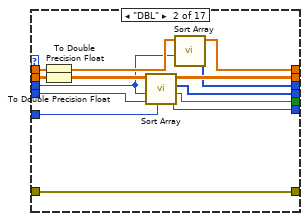
[diagram p3: hidden frame]
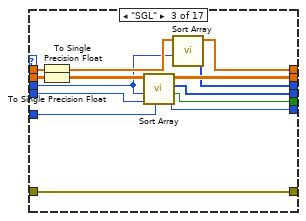
[diagram p4: hidden frame]
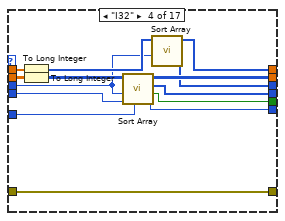
[diagram p5: hidden frame]
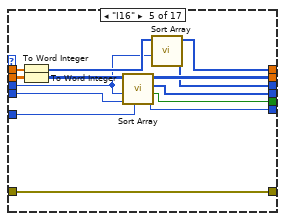
[diagram p6: hidden frame]
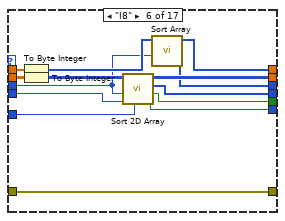
[diagram p7: hidden frame]
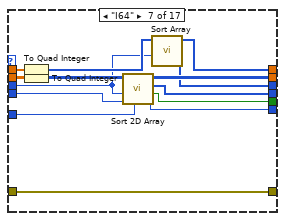
[diagram p8: hidden frame]
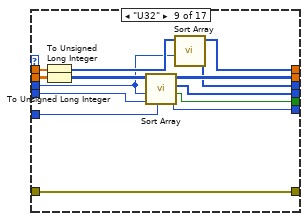
[diagram p9: hidden frame]
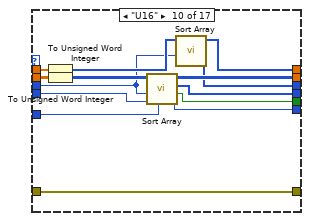
[diagram p10: hidden frame]
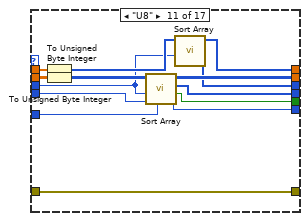
[diagram p11: hidden frame]
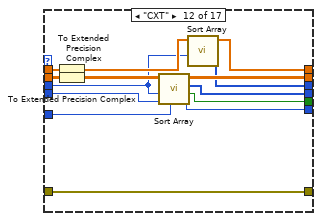
[diagram p12: hidden frame]
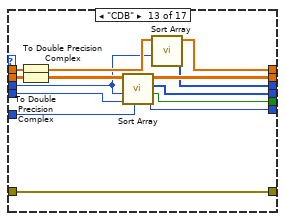
[diagram p13: hidden frame]
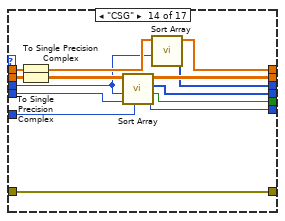
[diagram p14: hidden frame]
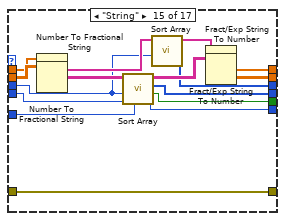
[diagram p15: hidden frame]
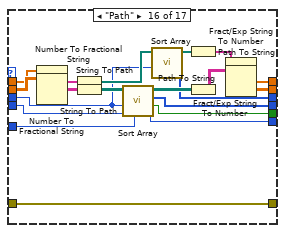
[diagram p16: hidden frame]
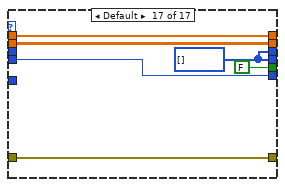
[diagram p17: hidden frame]
diagram:
  n1 = case shown="No Error" "error in (no error)" {
    selector: "error in (no error)" -> [w16 w286]
    tunnel: [w17 w286] -> w6
    tunnel: "Expected Outputs" -> [w14 _]
    tunnel: "Inputs" -> [w15 _]
    tunnel: [w13 _] -> w3
    tunnel: [w12 _] -> w1
    frame No Error {
      n2 = for {
        shift-right: [w25] -> w17
        shift-left: w16 -> [w26]
        tunnel: w15 -> [w27] mode=indexing
        tunnel: w14 -> [w30] mode=indexing
        tunnel: [w29] -> w13 mode=indexing
        tunnel: [w24] -> w11 mode=indexing
        n3 = Unbundle(w27) -> ("Data Types to Test"=w22:T3[], "1D Array"=w20:sgl[], "2D Array"=w21:sgl[][], "Order"=w19:enum16{"ascending", "descending"}, "Sort By in"=w18:enum16{"row", "column"}, "Column/Row to Sort By"=w23:u32)  [unwired: 1 out]
        n4 = for {
          tunnel: w30 -> [w47]
          tunnel: [w45] -> w29 mode=indexing
          tunnel: [w46] -> w28 mode=indexing
          shift-right: [w40] -> w25
          shift-left: w26 -> [w41]
          tunnel: w22 -> [w42] mode=indexing
          tunnel: w20 -> [w44]
          tunnel: w21 -> [w43]
          tunnel: w23 -> [w37]
          tunnel: w19 -> [w36]
          tunnel: w18 -> [w35]
          n5 = case shown="\"U64\"" w42 {
            tunnel: w44 -> [w60 w74 w88 w102 w116 w130 w144 w158 w172 w186 w200 w214 w228 w242 w258 w276 w284]
            tunnel: [w57 w71 w85 w99 w113 w127 w141 w155 w169 w183 w197 w211 w225 w239 w252 w269 w284] -> w39
            tunnel: [w56 w70 w84 w98 w112 w126 w140 w154 w168 w182 w196 w210 w224 w238 w251 w270 w283] -> w38
            tunnel: w43 -> [w61 w75 w89 w103 w117 w131 w145 w159 w173 w187 w201 w215 w229 w243 w259 w278 w283]
            tunnel: w41 -> [w58 w72 w86 w100 w114 w128 w142 w156 w170 w184 w198 w212 w226 w240 w257 w275 w285]
            tunnel: [w58 w72 w86 w100 w114 w128 w142 w156 w170 w184 w198 w212 w226 w240 w257 w275 w285] -> w40
            tunnel: w37 -> [w52 w67 w82 w96 w110 w122 w136 w150 w164 w180 w192 w206 w222 w236 w248 w264 _]
            tunnel: w36 -> [w54 w68 w81 w95 w109 w124 w138 w152 w166 w179 w194 w208 w221 w235 w250 w265 _]
            tunnel: w35 -> [w53 w66 w80 w94 w108 w123 w137 w151 w165 w178 w193 w207 w220 w234 w249 w266 w280]
            tunnel: [w50 w64 w78 w92 w106 w120 w134 w148 w162 w176 w190 w204 w219 w232 w246 w262 w282] -> w34
            tunnel: [w51 w65 w79 w93 w107 w121 w135 w149 w163 w177 w191 w205 w218 w233 w247 w263 w282] -> w33
            tunnel: [w49 w63 w77 w91 w105 w119 w133 w147 w161 w175 w189 w203 w217 w231 w245 w261 FALSE ("Index Out of Range?")] -> w32
            tunnel: [w48 w62 w76 w90 w104 w118 w132 w146 w160 w174 w188 w202 w216 w230 w244 w260 w280] -> w31
            frame "EXT" {
              n6 = To Extended Precision Float(1:w60) -> (0:w59:ext[])
              n7 = To Extended Precision Float(1:w61) -> (0:w55:ext[][])
              n8 = call-poly "Sort Array.vi"("Column/Row to Sort By"=w52, "Sort By in"=w53, "Order"=w54, "Array in"=w55) -> ("Sort By out"=w48:enum16{"row", "column"}, "Index Out of Range?"=w49:bool, "Sorted Pointers"=w50:i32[], "Sorted Array out"=w56:ext[][])  [unwired: 4 in]
              n9 = call-poly "Sort Array.vi"("Order"=w54, "Array in"=w59) -> ("Sorted Pointers"=w51:i32[], "Sorted Array out"=w57:ext[])  [unwired: 8 in]
            }
            frame "DBL" {
              n10 = To Double Precision Float(number=w74) -> (double precision float=w73:dbl[])
              n11 = To Double Precision Float(number=w75) -> (double precision float=w69:dbl[][])
              n12 = call-poly "Sort Array.vi"("Column/Row to Sort By"=w67, "Sort By in"=w66, "Order"=w68, "Array in"=w69) -> ("Sort By out"=w62:enum16{"row", "column"}, "Index Out of Range?"=w63:bool, "Sorted Pointers"=w64:i32[], "Sorted Array out"=w70:dbl[][])  [unwired: 4 in]
              n13 = call-poly "Sort Array.vi"("Order"=w68, "Array in"=w73) -> ("Sorted Pointers"=w65:i32[], "Sorted Array out"=w71:dbl[])  [unwired: 8 in]
            }
            frame "SGL" {
              n14 = To Single Precision Float(number=w88) -> (single precision float=w87:sgl[])
              n15 = To Single Precision Float(number=w89) -> (single precision float=w83:sgl[][])
              n16 = call-poly "Sort Array.vi"("Column/Row to Sort By"=w82, "Sort By in"=w80, "Order"=w81, "Array in"=w83) -> ("Sort By out"=w76:enum16{"row", "column"}, "Index Out of Range?"=w77:bool, "Sorted Pointers"=w78:i32[], "Sorted Array out"=w84:sgl[][])  [unwired: 4 in]
              n17 = call-poly "Sort Array.vi"("Order"=w81, "Array in"=w87) -> ("Sorted Pointers"=w79:i32[], "Sorted Array out"=w85:sgl[])  [unwired: 8 in]
            }
            frame "I32" {
              n18 = To Long Integer(number=w102) -> (32bit integer=w101:i32[])
              n19 = To Long Integer(number=w103) -> (32bit integer=w97:i32[][])
              n20 = call-poly "Sort Array.vi"("Column/Row to Sort By"=w96, "Sort By in"=w94, "Order"=w95, "Array in"=w97) -> ("Sort By out"=w90:enum16{"row", "column"}, "Index Out of Range?"=w91:bool, "Sorted Pointers"=w92:i32[], "Sorted Array out"=w98:i32[][])  [unwired: 4 in]
              n21 = call-poly "Sort Array.vi"("Order"=w95, "Array in"=w101) -> ("Sorted Pointers"=w93:i32[], "Sorted Array out"=w99:i32[])  [unwired: 8 in]
            }
            frame "I16" {
              n22 = To Word Integer(number=w116) -> (16bit integer=w115:i16[])
              n23 = To Word Integer(number=w117) -> (16bit integer=w111:i16[][])
              n24 = call-poly "Sort Array.vi"("Column/Row to Sort By"=w110, "Sort By in"=w108, "Order"=w109, "Array in"=w111) -> ("Sort By out"=w104:enum16{"row", "column"}, "Index Out of Range?"=w105:bool, "Sorted Pointers"=w106:i32[], "Sorted Array out"=w112:i16[][])  [unwired: 4 in]
              n25 = call-poly "Sort Array.vi"("Order"=w109, "Array in"=w115) -> ("Sorted Pointers"=w107:i32[], "Sorted Array out"=w113:i16[])  [unwired: 8 in]
            }
            frame "I8" {
              n26 = To Byte Integer(number=w130) -> (8bit integer=w129:i8[])
              n27 = To Byte Integer(number=w131) -> (8bit integer=w125:i8[][])
              n28 = call-poly "Sort 2D Array.vi"("Column/Row to Sort By"=w122, "Sort By in"=w123, "Order"=w124, "Array in"=w125) -> ("Sort By out"=w118:enum16{"row", "column"}, "Index Out of Range?"=w119:bool, "Sorted Pointers"=w120:i32[], "Sorted Array out"=w126:i8[][])  [unwired: 4 in]
              n29 = call-poly "Sort Array.vi"("Order"=w124, "Array in"=w129) -> ("Sorted Pointers"=w121:i32[], "Sorted Array out"=w127:i8[])  [unwired: 8 in]
            }
            frame "I64" {
              n30 = To Quad Integer(1:w144) -> (0:w143:i64[])
              n31 = To Quad Integer(1:w145) -> (0:w139:i64[][])
              n32 = call-poly "Sort 2D Array.vi"("Column/Row to Sort By"=w136, "Sort By in"=w137, "Order"=w138, "Array in"=w139) -> ("Sort By out"=w132:enum16{"row", "column"}, "Index Out of Range?"=w133:bool, "Sorted Pointers"=w134:i32[], "Sorted Array out"=w140:i64[][])  [unwired: 4 in]
              n33 = call-poly "Sort Array.vi"("Order"=w138, "Array in"=w143) -> ("Sorted Pointers"=w135:i32[], "Sorted Array out"=w141:i64[])  [unwired: 8 in]
            }
            frame "U64" {
              n34 = To Unsigned Quad Integer(1:w158) -> (0:w157:u64[])
              n35 = To Unsigned Quad Integer(1:w159) -> (0:w153:u64[][])
              n36 = call-poly "Sort 2D Array.vi"("Column/Row to Sort By"=w150, "Sort By in"=w151, "Order"=w152, "Array in"=w153) -> ("Sort By out"=w146:enum16{"row", "column"}, "Index Out of Range?"=w147:bool, "Sorted Pointers"=w148:i32[], "Sorted Array out"=w154:u64[][])  [unwired: 4 in]
              n37 = call-poly "Sort Array.vi"("Order"=w152, "Array in"=w157) -> ("Sorted Pointers"=w149:i32[], "Sorted Array out"=w155:u64[])  [unwired: 8 in]
            }
            frame "U32" {
              n38 = To Unsigned Long Integer(number=w172) -> (unsigned 32bit integer=w171:u32[])
              n39 = To Unsigned Long Integer(number=w173) -> (unsigned 32bit integer=w167:u32[][])
              n40 = call-poly "Sort Array.vi"("Column/Row to Sort By"=w164, "Sort By in"=w165, "Order"=w166, "Array in"=w167) -> ("Sort By out"=w160:enum16{"row", "column"}, "Index Out of Range?"=w161:bool, "Sorted Pointers"=w162:i32[], "Sorted Array out"=w168:u32[][])  [unwired: 4 in]
              n41 = call-poly "Sort Array.vi"("Order"=w166, "Array in"=w171) -> ("Sorted Pointers"=w163:i32[], "Sorted Array out"=w169:u32[])  [unwired: 8 in]
            }
            frame "U16" {
              n42 = To Unsigned Word Integer(number=w186) -> (unsigned 16bit integer=w185:u16[])
              n43 = To Unsigned Word Integer(number=w187) -> (unsigned 16bit integer=w181:u16[][])
              n44 = call-poly "Sort Array.vi"("Column/Row to Sort By"=w180, "Sort By in"=w178, "Order"=w179, "Array in"=w181) -> ("Sort By out"=w174:enum16{"row", "column"}, "Index Out of Range?"=w175:bool, "Sorted Pointers"=w176:i32[], "Sorted Array out"=w182:u16[][])  [unwired: 4 in]
              n45 = call-poly "Sort Array.vi"("Order"=w179, "Array in"=w185) -> ("Sorted Pointers"=w177:i32[], "Sorted Array out"=w183:u16[])  [unwired: 8 in]
            }
            frame "U8" {
              n46 = To Unsigned Byte Integer(number=w200) -> (unsigned 8bit integer=w199:u8[])
              n47 = To Unsigned Byte Integer(number=w201) -> (unsigned 8bit integer=w195:u8[][])
              n48 = call-poly "Sort Array.vi"("Column/Row to Sort By"=w192, "Sort By in"=w193, "Order"=w194, "Array in"=w195) -> ("Sort By out"=w188:enum16{"row", "column"}, "Index Out of Range?"=w189:bool, "Sorted Pointers"=w190:i32[], "Sorted Array out"=w196:u8[][])  [unwired: 4 in]
              n49 = call-poly "Sort Array.vi"("Order"=w194, "Array in"=w199) -> ("Sorted Pointers"=w191:i32[], "Sorted Array out"=w197:u8[])  [unwired: 8 in]
            }
            frame "CXT" {
              n50 = To Extended Precision Complex(1:w214) -> (0:w213:cxt[])
              n51 = To Extended Precision Complex(1:w215) -> (0:w209:cxt[][])
              n52 = call-poly "Sort Array.vi"("Column/Row to Sort By"=w206, "Sort By in"=w207, "Order"=w208, "Array in"=w209) -> ("Sort By out"=w202:enum16{"row", "column"}, "Index Out of Range?"=w203:bool, "Sorted Pointers"=w204:i32[], "Sorted Array out"=w210:cxt[][])  [unwired: 4 in]
              n53 = call-poly "Sort Array.vi"("Order"=w208, "Array in"=w213) -> ("Sorted Pointers"=w205:i32[], "Sorted Array out"=w211:cxt[])  [unwired: 8 in]
            }
            frame "CDB" {
              n54 = To Double Precision Complex(1:w228) -> (0:w227:cdb[])
              n55 = To Double Precision Complex(1:w229) -> (0:w223:cdb[][])
              n56 = call-poly "Sort Array.vi"("Column/Row to Sort By"=w222, "Sort By in"=w220, "Order"=w221, "Array in"=w223) -> ("Sort By out"=w216:enum16{"row", "column"}, "Index Out of Range?"=w217:bool, "Sorted Pointers"=w219:i32[], "Sorted Array out"=w224:cdb[][])  [unwired: 4 in]
              n57 = call-poly "Sort Array.vi"("Order"=w221, "Array in"=w227) -> ("Sorted Pointers"=w218:i32[], "Sorted Array out"=w225:cdb[])  [unwired: 8 in]
            }
            frame "CSG" {
              n58 = To Single Precision Complex(1:w242) -> (0:w241:csg[])
              n59 = To Single Precision Complex(1:w243) -> (0:w237:csg[][])
              n60 = call-poly "Sort Array.vi"("Column/Row to Sort By"=w236, "Sort By in"=w234, "Order"=w235, "Array in"=w237) -> ("Sort By out"=w230:enum16{"row", "column"}, "Index Out of Range?"=w231:bool, "Sorted Pointers"=w232:i32[], "Sorted Array out"=w238:csg[][])  [unwired: 4 in]
              n61 = call-poly "Sort Array.vi"("Order"=w235, "Array in"=w241) -> ("Sorted Pointers"=w233:i32[], "Sorted Array out"=w239:csg[])  [unwired: 8 in]
            }
            frame "String" {
              n62 = Number To Fractional String(number=w258) -> (F-format string=w256:string[])  [unwired: 3 in]
              n63 = Number To Fractional String(number=w259) -> (F-format string=w255:string[][])  [unwired: 3 in]
              n64 = call-poly "Sort Array.vi"("Column/Row to Sort By"=w248, "Sort By in"=w249, "Order"=w250, "Array in"=w255) -> ("Sort By out"=w244:enum16{"row", "column"}, "Index Out of Range?"=w245:bool, "Sorted Pointers"=w246:i32[], "Sorted Array out"=w253:string[][])  [unwired: 4 in]
              n65 = call-poly "Sort Array.vi"("Order"=w250, "Array in"=w256) -> ("Sorted Pointers"=w247:i32[], "Sorted Array out"=w254:string[])  [unwired: 8 in]
              n66 = Fract/Exp String To Number(string=w254) -> (number=w252:dbl[])  [unwired: 3 in, 1 out]
              n67 = Fract/Exp String To Number(string=w253) -> (number=w251:dbl[][])  [unwired: 3 in, 1 out]
            }
            frame "Path" {
              n68 = Number To Fractional String(number=w276) -> (F-format string=w277:string[])  [unwired: 3 in]
              n69 = Number To Fractional String(number=w278) -> (F-format string=w279:string[][])  [unwired: 3 in]
              n70 = String To Path(string=w277) -> (path=w274:path[])
              n71 = String To Path(string=w279) -> (path=w271:path[][])
              n72 = call-poly "Sort Array.vi"("Column/Row to Sort By"=w264, "Sort By in"=w266, "Order"=w265, "Array in"=w271) -> ("Sort By out"=w260:enum16{"row", "column"}, "Index Out of Range?"=w261:bool, "Sorted Pointers"=w262:i32[], "Sorted Array out"=w272:path[][])  [unwired: 4 in]
              n73 = call-poly "Sort Array.vi"("Order"=w265, "Array in"=w274) -> ("Sorted Pointers"=w263:i32[], "Sorted Array out"=w273:path[])  [unwired: 8 in]
              n74 = Path To String(path=w273) -> (string=w268:string[])
              n75 = Path To String(path=w272) -> (string=w267:string[][])
              n76 = Fract/Exp String To Number(string=w268) -> (number=w269:dbl[])  [unwired: 3 in, 1 out]
              n77 = Fract/Exp String To Number(string=w267) -> (number=w270:dbl[][])  [unwired: 3 in, 1 out]
            }
            frame Default {
              w282 = i32[] [] ("Sorted Pointers")
            }
          }
          n78 = Bundle(cluster=w47, "1D Array"=w39, "2D Array"=w38, "1D Sorted Pointers"=w33, "2D Sorted Pointers"=w34, "Index Out of Range?"=w32, "Sort By in"=w31) -> (w45:T1)  [unwired: 1 in]
          n79 = Equal?(x=w47, y=w45) -> (x = y?=w46:bool)
        }
        n80 = And Array Elements(Boolean array=w28) -> (logical AND=w24:bool)
      }
      n81 = Search 1D Array(1D array=w11, element=FALSE) -> (index of element=w9:i32)  [unwired: 1 in]
      n82 = And Array Elements(Boolean array=w11) -> (logical AND=w12:bool)
      n83 = Build Array(w9) -> (w8:i32[])
      n84 = property on="Inputs" class="Arr (strict)"("Index Values"=w8) -> ()  [unwired: 2 in, 2 out]
      n85 = property on="Expected Outputs" class="Arr (strict)"("Index Values"=w8) -> ()  [unwired: 2 in, 2 out]
      n86 = property on="Generated Outputs" class="Arr (strict)"("Index Values"=w8) -> ()  [unwired: 2 in, 2 out]
    }
    frame Error {
    }
  }
  "error out" <- w6
  "Pass?" <- w1
  "Generated Outputs" <- w3
  n87 = Not(x=w1) -> (.not. x?=w2:bool)
  n88 = call "Open Caller's Front Panel.vi"("Open?"=w2) -> ()  [unwired: 14 in, 1 out]
